vi "Z6_Beamline.set GUI Refs.vi"(0 "VI in":refnum<vi>, 1 "Class":string, 2 "Z6 Beamline GUI Refs":T3, 3 "PH_BL_Master GUI Refs":T1, 4 "System Information GUI Refs":T2, 5 "error in (no error)":errorcluster) -> (14 "VI out":refnum<vi>, 19 "error out":errorcluster)   [LabVIEW 2014, in "Z6_Beamline.lvlib"]
uses:
  Z6_Beamline.lvlib
  Z6_Beamline.GUI Refs.ctl
  Z6_Beamline.Subsystem ok GUI Refs.ctl
  PH_SystemInformation/PH_SystemInformation.GUI Refs.ctl
  PH_BL-Master/PH_BL-Master.GUI Refs.ctl
  PH_BL-Master/PH_BL-Master.lvlib
  PH_SystemInformation/PH_SystemInformation.lvlib
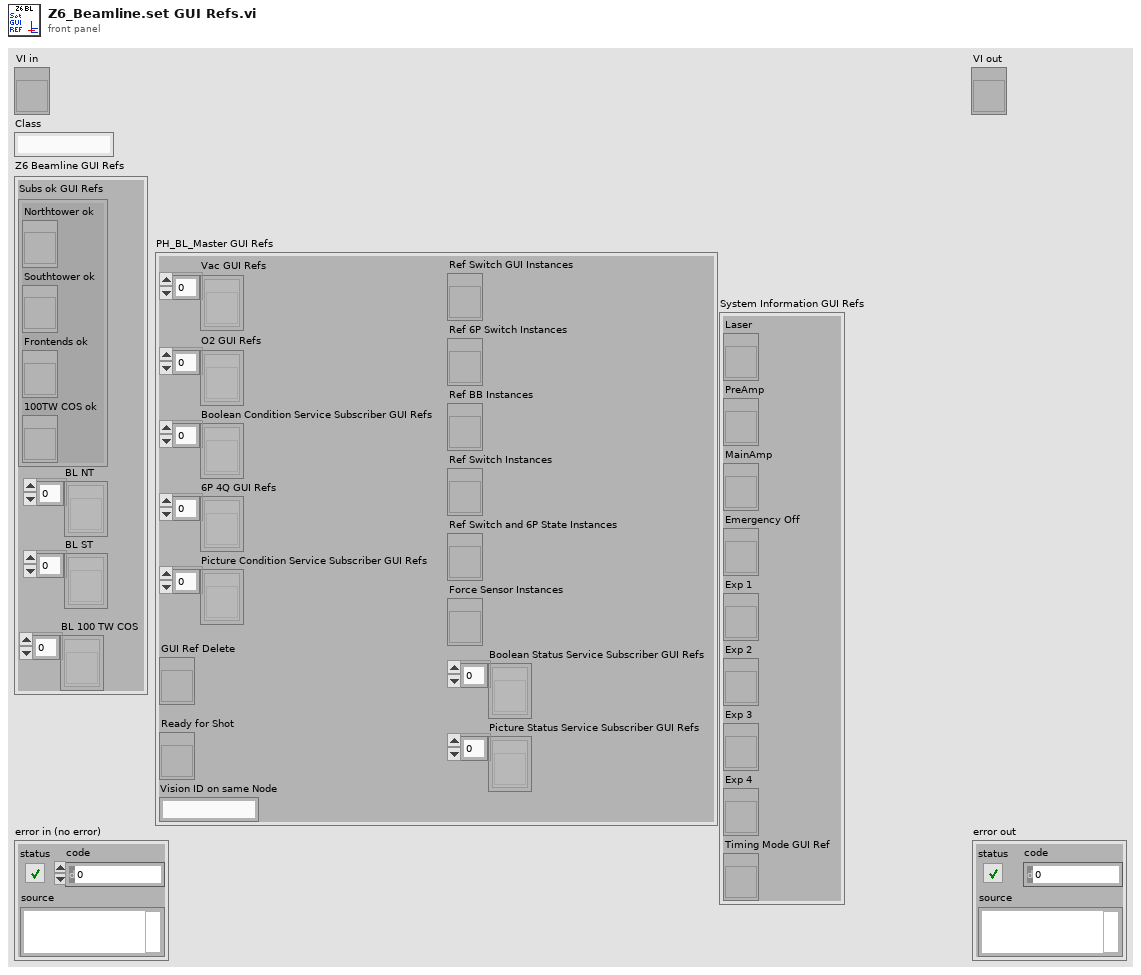
[diagram p1: front panel]
types:
  T1 = typedef "PH_BL-Master.lvlib/PH_BL-Master.GUI Refs.ctl" = cluster{"Vac GUI Refs":refnum<vi>[], "O2 GUI Refs":refnum<vi>[], "Ready for Shot":refnum<vi>, "Boolean Condition Service Subscriber GUI Refs":refnum<vi>[], "Vision ID on same Node":string, "Picture Condition Service Subscriber GUI Refs":refnum<vi>[], "6P 4Q GUI Refs":refnum<vi>[], "Ref Switch GUI Instances":refnum<vi>, "Ref 6P Switch Instances":refnum<vi>, "Ref BB Instances":refnum<vi>, "Ref Switch Instances":refnum<vi>, "Ref Switch and 6P State Instances":refnum<vi>, "Boolean Status Service Subscriber GUI Refs":refnum<vi>[], "Picture Status Service Subscriber GUI Refs":refnum<vi>[], "Force Sensor Instances":refnum<vi>, "GUI Ref Delete":refnum<vi>}
  T2 = typedef "PH_SystemInformation.lvlib/PH_SystemInformation.GUI Refs.ctl" = cluster{"Laser":refnum<vi>, "PreAmp":refnum<vi>, "MainAmp":refnum<vi>, "Emergency Off":refnum<vi>, "Exp 1":refnum<vi>, "Exp 2":refnum<vi>, "Exp 3":refnum<vi>, "Exp 4":refnum<vi>, "Timing Mode GUI Ref":refnum<vi>}
  T3 = typedef "Z6_Beamline.lvlib/Z6_Beamline.GUI Refs.ctl" = cluster{"BL NT":refnum<vi>[], "BL ST":refnum<vi>[], "BL 100 TW COS":refnum<vi>[], "Subs ok GUI Refs":T4}
  T4 = typedef "Z6_Beamline.lvlib/Z6_Beamline.Subsystem ok GUI Refs.ctl" = cluster{"Northtower ok":refnum<vi>, "Southtower ok":refnum<vi>, "Frontends ok":refnum<vi>, "100TW COS ok":refnum<vi>}
  T5 = typedef "Z6_Beamline.lvlib/Z6_Beamline.i attribute.ctl" = cluster{"Subs ok GUI Refs":T4, "Refs BL Northtower":refnum<vi>[], "Refs BL Southtower":refnum<vi>[], "Refs BL 100TW COS":refnum<vi>[], "State Subsystems":cluster{"Northtower":bool, "Southtower":bool, "Frontends":bool, "100TW COS":bool}, "Z6 Beamline Status Subscriber Information":T6, "Color State PHELIX":i16}
  T6 = typedef "Z6_Beamline.lvlib/Z6_Beamline.Status Subscriber Information.ctl" = cluster{"BL Z6 Shutter":T7, "CH 10":T7, "CH 11":T7, "ST Flip Cam":T7, "ST Flip DB":T7, "BL Z6 Dump":T7}
  T7 = typedef "PH_BL-Master.lvlib/PH_BL-Master.Status Subscriber Information.ctl" = cluster{"Index of element":i32, "Attributeset":T8}
  T8 = typedef "PH_BL-Master.lvlib/PH_BL-Master.Attribute Set.ctl" = enum16{"Boolean Status Service Subscriber", "Picture Status Service Subscriber"}
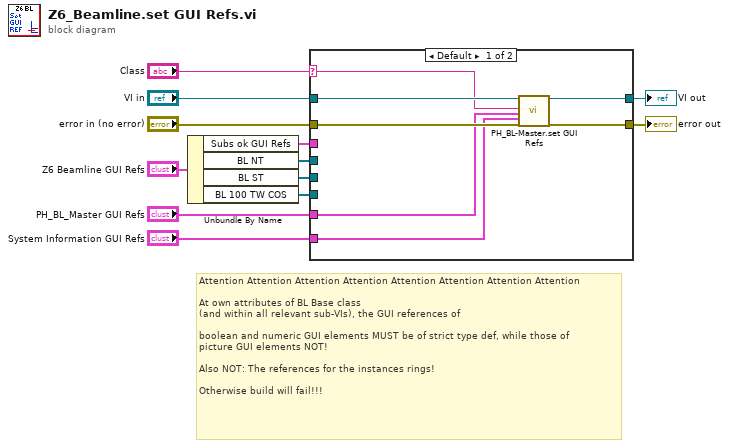
[diagram p0: block diagram]
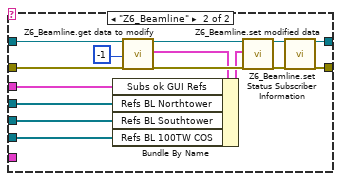
[diagram p2: hidden frame]
diagram:
  # "Attention Attention Attention Attention Attention Attention Attention Attention\n\nAt own attributes of BL Base class \n(and within all relevant sub-VIs), the GUI references of\n\nboolean and numeric GUI elements MUST be of strict type def, while those of\npicture GUI elements NOT!\n\nAlso NOT: The references for the instances rings!\n\nOtherwise build will fail!!!"
  n1 = Unbundle By Name("Z6 Beamline GUI Refs") -> ("Subs ok GUI Refs"=w6:T4, "BL NT"=w5:refnum<vi>[], "BL ST"=w4:refnum<vi>[], "BL 100 TW COS"=w3:refnum<vi>[])
  n2 = case shown="Default" "Class" {
    selector: "Class" -> [w15 _]
    tunnel: "VI in" -> [w17 w31]
    tunnel: [w16 w21] -> w12
    tunnel: "error in (no error)" -> [w19 w30]
    tunnel: [w18 w20] -> w10
    tunnel: w6 -> [_ w25]
    tunnel: w5 -> [_ w24]
    tunnel: w4 -> [_ w23]
    tunnel: w3 -> [_ w22]
    tunnel: "PH_BL_Master GUI Refs" -> [w14 _]
    tunnel: "System Information GUI Refs" -> [w13 _]
    frame Default {
      n3 = call "PH_BL-Master.set GUI Refs.vi"("i ref in"=w17, "Class"=w15, "PH_BL-Master GUI Refs"=w14, "System Information GUI Refs"=w13, "error in"=w19) -> ("i ref out"=w16:refnum<vi>, "error out"=w18:errorcluster)  [unwired: 13 in]
    }
    frame "Z6_Beamline" {
      n4 = call "Z6_Beamline.get data to modify.vi"("i ref in"=w31, "ms timeout (10000)"=-1, "error in (no error)"=w30) -> ("i ref out"=w34:refnum<vi>, "i attribute"=w27:T5, "error out"=w33:errorcluster)  [unwired: 13 in, 1 out]
      n5 = Bundle By Name(cluster=w27, "Subs ok GUI Refs"=w25, "Refs BL Northtower"=w24, "Refs BL Southtower"=w23, "Refs BL 100TW COS"=w22) -> (w26:T5)
      n6 = call "Z6_Beamline.set modified data.vi"("i ref in"=w34, "i attribute"=w26, "error in (no error)"=w33) -> ("i ref out"=w29:refnum<vi>, "error out"=w28:errorcluster)  [unwired: 15 in]
      n7 = call "Z6_Beamline.set Status Subscriber Information.vi"("i ref in"=w29, "error in (no error)"=w28) -> ("i ref out"=w21:refnum<vi>, "error out"=w20:errorcluster)  [unwired: 16 in]
    }
  }
  "VI out" <- w12
  "error out" <- w10
